vi "Create Slave Instance (Serial).vi"(4 "flow control (None)":u16(ring) items=["None", "XON/XOFF", "RTS/CTS", "XON/XOFF & RTS/CTS", "DTR/DSR", "XON/XOFF & DTR/DSR"], 5 "serial type":enum16{"RTU", "ASCII"}(ring), 6 "parity (Even)":u16(ring)=2 items=["None", "Odd", "Even"], 7 "unit ID":u8=1, 8 "error in (no error)":errorcluster, 9 "device data model":refnum<class "Device Data Model.lvclass">, 10 "baud rate (9600)":u32=9600, 11 "VISA resource name":refnum<visa-resource-name>) -> (0 "error out":errorcluster, 3 "serial slave instance":refnum<class "Modbus Slave.lvclass">)   [LabVIEW 2017, in "Modbus Slave.lvclass"]
doc: "Creates a serial or TCP Modbus slave instance. The Modbus slave instance you create includes a daemon. Daemon is a background process that responds to requests from Modbus master instances. You must manually select the polymorphic instance to use."
uses:
  <vilib>/Modbus/slave/Modbus Slave.lvclass
  C:/builds/penguin/iak/lvdsc/trunk/17.0/lv/vi.lib/Modbus/subvis/Modbus API/Modbus API.lvclass
  <vilib>/Modbus/subvis/Data and Functions/Device Data Model/Device Data Model.lvclass
  <vilib>/Modbus/subvis/Transmission Data Unit (ADU)/RTU Data Unit/RTU Data Unit.lvclass
  C:/builds/penguin/iak/lvdsc/trunk/17.0/lv/vi.lib/Modbus/subvis/Transmission Data Unit (ADU)/Serial Data Unit/Serial Data Unit.lvclass
  <vilib>/Modbus/subvis/Transmission Data Unit (ADU)/ASCII Data Unit/ASCII Data Unit.lvclass
  <vilib>/Modbus/subvis/Transmission Data Unit (ADU)/Transmission Data Unit/Transmission Data Unit.lvclass/Transmission Data Unit.ctl
  <vilib>/Modbus/subvis/Protocol/Serial/Serial Slave/Serial Slave.lvclass
  C:/builds/penguin/iak/lvdsc/trunk/17.0/lv/vi.lib/Modbus/subvis/Protocol/Interfaces/Network Slave/Network Slave.lvclass
  <vilib>/Modbus/subvis/Data and Functions/Standard Data Model/Standard Data Model.lvclass
  C:/builds/penguin/iak/lvdsc/trunk/17.0/lv/vi.lib/Modbus/subvis/Data and Functions/Device Data Model/Device Data Model.lvclass
  <vilib>/Modbus/subvis/Data and Functions/Device Data Model/Device Data Model.lvclass/Device Data Model.ctl
  <vilib>/Modbus/subvis/Protocol/Serial/Serial Slave/Serial Slave.lvclass/Serial Slave.ctl
  <vilib>/Modbus/slave/Modbus Slave.lvclass/Modbus Slave.ctl
  <vilib>/Modbus/subvis/Modbus API/Modbus API.lvclass/Modbus API.ctl
  <vilib>/Modbus/subvis/Protocol/Serial/Serial Slave/Data Access/Baud Rate/Write Baud Rate.vi
  <vilib>/Modbus/subvis/Protocol/Serial/Serial Slave/Data Access/Flow Control/Write Flow Control.vi
  <vilib>/Modbus/subvis/Protocol/Serial/Serial Slave/Data Access/Parity/Write Parity.vi
  <vilib>/Modbus/subvis/Protocol/Serial/Serial Slave/Data Access/VISA resource name/Write VISA resource name.vi
  <vilib>/Modbus/subvis/Protocol/Serial/Serial Slave/Data Access/Serial Data Unit/Write Serial Data Unit.vi
  <vilib>/Modbus/subvis/Data and Functions/Device Data Model/Data Access/Initialized/Read Initialized.vi
  <vilib>/Utility/error.llb/Clear Errors.vi
  <vilib>/Modbus/subvis/Transmission Data Unit (ADU)/Serial Data Unit/Serial Data Unit.lvclass
  C:/builds/penguin/iak/lvdsc/trunk/17.0/lv/vi.lib/Modbus/subvis/Transmission Data Unit (ADU)/Transmission Data Unit/Transmission Data Unit.lvclass
  <vilib>/Modbus/subvis/Modbus API/Modbus API.lvclass
  <vilib>/Modbus/subvis/Transmission Data Unit (ADU)/Transmission Data Unit/Transmission Data Unit.lvclass
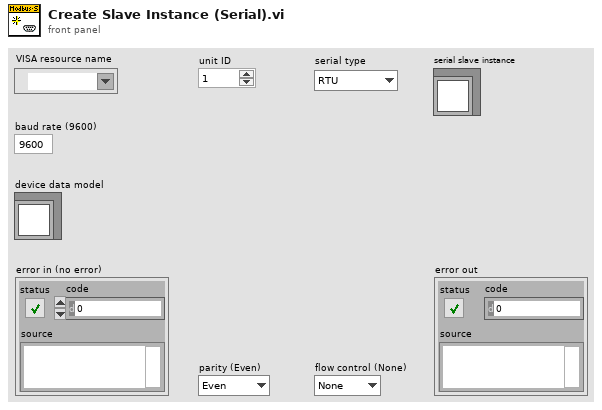
[diagram p1: front panel]
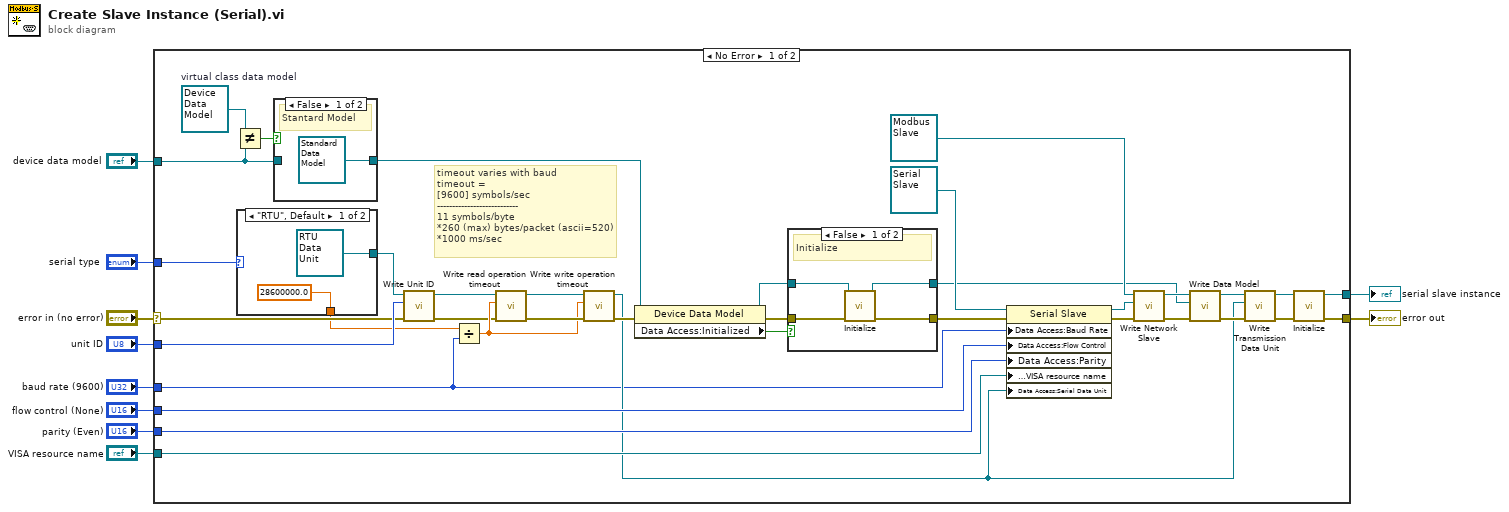
[diagram p0: block diagram]
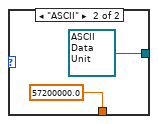
[diagram p4: hidden frame]
diagram:
  n1 = case shown="No Error" "error in (no error)" {
    selector: "error in (no error)" -> [w20 w60]
    tunnel: "VISA resource name" -> [w47 _]
    tunnel: [w46 w60] -> w9
    tunnel: "baud rate (9600)" -> [w12 _]
    tunnel: "flow control (None)" -> [w44 _]
    tunnel: "parity (Even)" -> [w43 _]
    tunnel: "serial type" -> [w42 _]
    tunnel: "device data model" -> [w36 _]
    tunnel: "unit ID" -> [w22 _]
    tunnel: [w21 _] -> w2
    frame No Error {
      w38 = refnum<class "Device Data Model.lvclass"> refnum  # virtual class data model
      # "timeout varies with baud\ntimeout =\n[9600] symbols/sec\n---------------------------\n11 symbols/byte\n*260 (max) bytes/packet (ascii=520)\n*1000 ms/sec"
      n2 = Not Equal?(x=w38, y=w36) -> (x != y?=w37:bool)
      n3 = case shown="\"RTU\", Default" w42 {
        tunnel: [refnum<class "RTU Data Unit.lvclass"> refnum ("RTU Data Unit") refnum<class "ASCII Data Unit.lvclass"> refnum ("ASCII Data Unit")] -> w23
        tunnel: [28600000.0 ("x") 57200000.0 ("x")] -> w11
        frame "RTU", Default {
        }
        frame "ASCII" {
        }
      }
      n4 = case shown="False" w37 {
        tunnel: w36 -> [_ w49]
        tunnel: [refnum<class "Standard Data Model.lvclass"> refnum ("Standard Data Model") w49] -> w34
        frame False {
          # "Stantard Model"
        }
        frame True {
        }
      }
      n5 = call <vilib>:"Write Unit ID.vi"("error in (no error)"=w20, "unit ID"=w22, "transmission data unit in"=w23) -> ("error out"=w15:errorcluster, "transmission data unit out"=w16:refnum<class "Serial Data Unit.lvclass">)  [unwired: 7 in]
      n6 = Divide(x=w11, y=w12) -> (x/y=w17:dbl)
      n7 = call <vilib>:"Write read operation timeout.vi"("error in (no error)"=w15, "read operation timeout"=w17, "transmission data unit in"=w16) -> ("error out"=w18:errorcluster, "transmission data unit out"=w19:refnum<class "Serial Data Unit.lvclass">)  [unwired: 7 in]
      n8 = call <vilib>:"Write write operation timeout.vi"("error in (no error)"=w18, "write operation timeout"=w17, "transmission data unit in"=w19) -> ("error out"=w14:errorcluster, "transmission data unit out"=w13:refnum<class "Serial Data Unit.lvclass">)  [unwired: 7 in]
      n9 = property class="Device Data Model"(reference=w34, error in=w14) -> (reference out=w40:refnum<class "Device Data Model.lvclass">, error out=w41:errorcluster, "Data Access:Initialized"=w39:bool)
      n10 = case shown="False" w39 {
        tunnel: w41 -> [w53 w55]
        tunnel: [w52 w55] -> w35
        tunnel: [w51 w54] -> w24
        tunnel: w40 -> [w50 w54]
        frame False {
          # "Initialize"
          n11 = call-dynamic "Initialize.vi"("error in (no error)"=w53, "device data model in"=w50) -> ("error out"=w52:errorcluster, "device data model out"=w51:refnum<class "Device Data Model.lvclass">)  [unwired: 8 in]
        }
        frame True {
        }
      }
      n12 = property class="Serial Slave"(reference=refnum<class "Serial Slave.lvclass"> refnum ("Serial Slave"), error in=w35, "Data Access:Baud Rate"=w12, "Data Access:Flow Control"=w44, "Data Access:Parity"=w43, "Data Access:VISA resource name"=w47, "Data Access:Serial Data Unit"=w13) -> (reference out=w29:refnum<class "Serial Slave.lvclass">, error out=w28:errorcluster)
      n13 = call <vilib>:"Write Network Slave.vi"("error in (no error)"=w28, "network slave"=w29, "Modbus slave in"=refnum<class "Modbus Slave.lvclass"> refnum ("Modbus Slave")) -> ("error out"=w27:errorcluster, "Modbus slave out"=w26:refnum<class "Modbus Slave.lvclass">)  [unwired: 7 in]
      n14 = call <vilib>:"Write Data Model.vi"("error in (no error)"=w27, "device data model"=w24, "Modbus slave in"=w26) -> ("error out"=w30:errorcluster, "Modbus slave out"=w31:refnum<class "Modbus Slave.lvclass">)  [unwired: 7 in]
      n15 = call <vilib>:"Write Transmission Data Unit.vi"("error in (no error)"=w30, "transmission data unit"=w13, "Modbus instance in"=w31) -> ("error out"=w32:errorcluster, "Modbus instance out"=w33:refnum<class "Modbus Slave.lvclass">)  [unwired: 7 in]
      n16 = call-dynamic "Initialize.vi"("error in (no error)"=w32, "Modbus slave in"=w33) -> ("error out"=w46:errorcluster, "Modbus slave out"=w21:refnum<class "Modbus Slave.lvclass">)  [unwired: 8 in]
    }
    frame Error {
    }
  }
  "error out" <- w9
  "serial slave instance" <- w2
